vi "NumberArray.140620.vi"   [LabVIEW 2013]
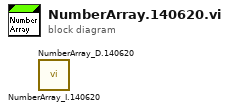
[diagram p0: block diagram]
diagram:
  n1 = call "NumberArray_I.140620.vi"() -> ()  [unwired: 10 in, 2 out]
  n2 = call "NumberArray_D.140620.vi"() -> ()  [unwired: 10 in, 2 out]
